vi "Get Write Setup.vi"(8 "error in (no error)":errorcluster, 11 "RxTx in":refnum<class "RxTx.lvclass">) -> (0 "error out":errorcluster, 3 "RxTx out":refnum<class "RxTx.lvclass">)   [LabVIEW 2018, in "RxTx.lvclass"]
uses:
  RxTx.lvclass
  RxTx.lvclass/RxTx.ctl
  Interface/Interface.lvclass
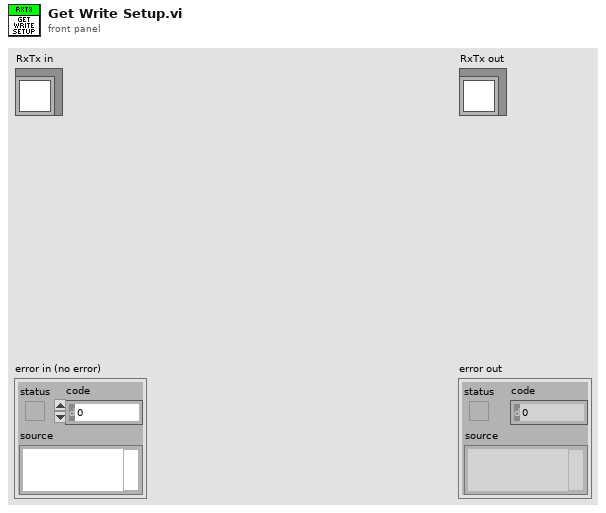
[diagram p1: front panel]
types:
  T1 = cluster{"EXPTIME":sgl, "PREAMP":u8, "READOUT_RATE":u8, "EM_MODE":u8, "EM_GAIN":u16, "BINNING":u16, "INITIAL_LINE":u16, "INITIAL_COLUMN":u16, "FINAL_LINE":u16, "FINAL_COLUMN":u16, "#FRAMES":u32, "SHUTTER_MODE":u8, "COOLER_POWER_STATUS":u16, "TEMP":i8, "#CUBES":u32, "TRIGGER_MODE":u16}
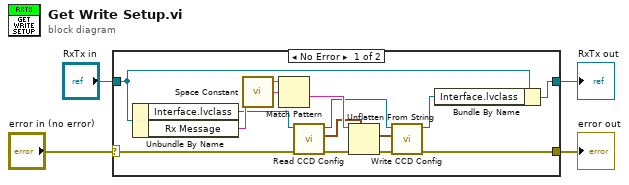
[diagram p0: block diagram]
diagram:
  n1 = case shown="No Error" "error in (no error)" {
    selector: "error in (no error)" -> [w10 w20]
    tunnel: [w14 w20] -> w2
    tunnel: [w12 w19] -> w1
    tunnel: "RxTx in" -> [w13 w19]
    frame No Error {
      n2 = Unbundle By Name(w13) -> ("Interface.lvclass"=w9:refnum<class "Interface.lvclass">, "Rx Message"=w15:string)
      n3 = call <vilib>:"Space Constant.vi"() -> ("String"=w18:string)
      n4 = Match Pattern(string=w15, regular expression=w18) -> (after substring=w17:string)  [unwired: 1 in, 3 out]
      n5 = call "Read CCD Config.vi"("error in (no error)"=w10, "Interface in"=w9) -> ("error out"=w6:errorcluster, "CCD Config"=w7:T1, "Interface out"=w8:refnum<class "Interface.lvclass">)  [unwired: 7 in]
      n6 = Unflatten From String(type=w7, binary string=w17, error in (no error)=w6) -> (value=w5:T1, error out=w11:errorcluster)  [unwired: 2 in, 1 out]
      n7 = call "Write CCD Config.vi"("error in (no error)"=w11, "CCD Config"=w5, "Interface in"=w8) -> ("error out"=w14:errorcluster, "Interface out"=w16:refnum<class "Interface.lvclass">)  [unwired: 7 in]
      n8 = Bundle By Name(cluster=w13, "Interface.lvclass"=w16) -> (w12:refnum<class "RxTx.lvclass">)
    }
    frame Error {
    }
  }
  "error out" <- w2
  "RxTx out" <- w1
